vi "Next Identity.vi"(7 "Previous In":refnum<class "Agent Identity.lvclass">, 8 "Error In":errorcluster, 10 "Next In":refnum<class "Agent Identity.lvclass">, 11 "Agent In":refnum<class "Agent.lvclass">) -> (0 "Error Out":errorcluster, 1 "Result":T1 items=["Success", "End of Identities"], 2 "Next Out":refnum<class "Agent Identity.lvclass">, 3 "Agent Out":refnum<class "Agent.lvclass">, 5 "Previous Out":refnum<class "Agent Identity.lvclass">)   [LabVIEW 2021, in "Field_RnD_Services_LIBSSH2_Toolkit.lvlib" / "Agent.lvclass"]
doc: "Gets the next identity in the internal libssh2lv shared library linked list of identities obtained from a SSH-agent application. Identities are obtained as a libssh2lv shared library internal linked list. This VI should be called after the first identity is retrieved, but it is safe to call in a loop to obtain all of the identities."
uses:
  Agent.lvclass
  Type Definitions/Results.ctl
  Agent Identity/Agent Identity.lvclass
  Agent.lvclass/Agent.ctl
  Field_RnD_Services_LIBSSH2_Toolkit.lvlib
  Session/Session.lvclass
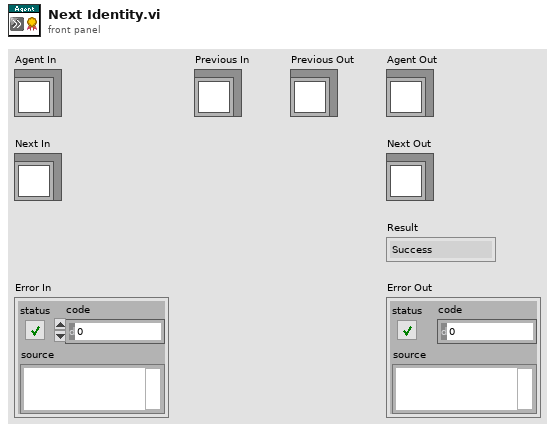
[diagram p1: front panel]
types:
  T1 = typedef "Field_RnD_Services_LIBSSH2_Toolkit.lvlib/Agent.lvclass/Results.ctl" = i32
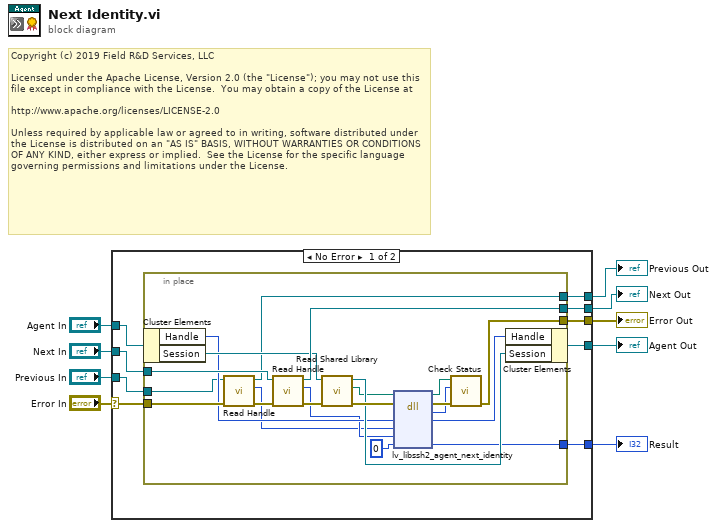
[diagram p0: block diagram]
diagram:
  # "Copyright (c) 2019 Field R&D Services, LLC\n\nLicensed under the Apache License, Version 2.0 (the \"License\"); you may not use this file except in compliance with the License.  You may obtain a copy of the License at\n\nhttp://www.apache.org/licenses/LICENSE-2.0\n\nUnless required by applicable law or agreed to in writing, software distributed under the License is distributed on an \"AS IS\" BASIS, WITHOUT WARRANTIES OR CONDITIONS OF ANY KIND, either express or implied.  See the License for the specific language governing permissions and limitations under the License."
  n1 = case shown="No Error" "Error In" {
    selector: "Error In" -> [w18 w43]
    tunnel: [w17 w43] -> w8
    tunnel: "Agent In" -> [w16 w42]
    tunnel: [w12 w42] -> w6
    tunnel: "Next In" -> [w15 w41]
    tunnel: [w14 w41] -> w4
    tunnel: "Previous In" -> [w13 w40]
    tunnel: [w11 w40] -> w2
    tunnel: [w10 _] -> w1
    frame No Error {
      n2 = in-place {
        in-place-border: w18 -> [w27]
        in-place-border: [w36] -> w17
        in-place-border: w15 -> [w30]
        in-place-border: [w28] -> w14
        in-place-border: w13 -> [w21]
        in-place-border: [w20] -> w11
        in-place-border: [w19] -> w10
        n3 = in-place-cluster #1(w16) -> ("Handle"=w25:u64, "Session"=w26:refnum<class "Session.lvclass">)
        n4 = call "Read Handle.vi"("Error In"=w27, "Identity In"=w21) -> ("Error Out"=w24:errorcluster, "Handle"=w22:u64, "Identity Out"=w20:refnum<class "Agent Identity.lvclass">)  [unwired: 7 in]
        n5 = call "Read Handle.vi"("Error In"=w24, "Identity In"=w30) -> ("Error Out"=w29:errorcluster, "Handle"=w23:u64, "Identity Out"=w28:refnum<class "Agent Identity.lvclass">)  [unwired: 7 in]
        n6 = call "Read Shared Library.vi"("Error In"=w29, "Session In"=w26) -> ("Erorr Out"=w34:errorcluster, "libssh2lv Shared Library"=w32:path, "Session Out"=w33:refnum<class "Session.lvclass">)  [unwired: 7 in]
        n7 = dll-call lib="libssh2lv.*" fn="lv_libssh2_agent_next_identity"(path in=w32, error in=w34, "handle"=w25, "previous"=w22, "next"=w23, "result"=0) -> (path out=w37:path, error out=w38:errorcluster, "status"=w35:i32, "handle"=w39:u64, "result"=w19:i32)  [unwired: 3 in]
        n8 = call "Check Status.vi"("Error In"=w38, "Status"=w35, "libssh2lv Shared Library In"=w37) -> ("Error Out"=w36:errorcluster)  [unwired: 7 in, 1 out]
        n9 = in-place-cluster #1("Handle"=w39, "Session"=w33) -> (w12:refnum<class "Agent.lvclass">)
      }
    }
    frame Error {
    }
  }
  "Error Out" <- w8
  "Result" <- w1
  "Agent Out" <- w6
  "Next Out" <- w4
  "Previous Out" <- w2
